vi "Monitor.vi"(8 "error in (no error)":errorcluster) -> ()   [LabVIEW 2015]
uses:
  <vilib>/Rock Robotics/Network Tables/NT Write Number.vi
  Utilities/MotorPositionGlobals.vi
  Utilities/GlobalVisionVars.vi
  MonitorGlobals.vi
  Utilities/ShiftGlobals.vi
  navx-mxp/labview/navX Library v2/navX Library v2.lvlib
panel:
  out "YRPHfH":T1
  out "Applied Throttle 2":dbl
  out "Applied Throttle":dbl
  out "Climber Current":dbl
  out "Climber Velocity":dbl
  out "Climber Position":dbl
  in  "Tab Control":enum32{"Position", "Vision Code", "Currents"}(tab)
  out "ArmMotor Encoder Position":dbl
  out "TensionerMotor Encoder Position":dbl
  out "WinchMotor Encoder Position":dbl
  out "WinchSetpoint":dbl
  out "TensionerSetpoint":dbl
  out "ArmSetpoint":dbl=195.0
  out "Manipulator Encoder":dbl
  out "Manipulator Setpoint":dbl
  out "Left Drive Encoder":dbl
  out "Right Drive Encoder":dbl
  out "Left Drive Velocity":dbl
  out "Right Drive Velocity":dbl
  out "Tensioner Limit Switch Pressed":bool
  out "Horizontal Gyro Angle":dbl
  out "LeftDriveError":dbl
  out "RightDriveError":dbl
  out "Heading vs Actual":dynamicdata(graph)
  out "TargetDistance":dbl
  out "Heading":dbl
  out "NumberOfParticles":i32
  out "OnTarget":bool
  out "Left1 Current":dbl
  out "Left2 Current":dbl
  out "Right1 Current":dbl
  out "Right2 Current":dbl
  out "Winch Current":dbl
  out "Arm Current":dbl
  out "Tensioner Current":dbl
  out "Manipulator Current":dbl
  out "all currents (A)":dbl[](array[numeric])
  out "Waveform Chart":dynamicdata(graph)
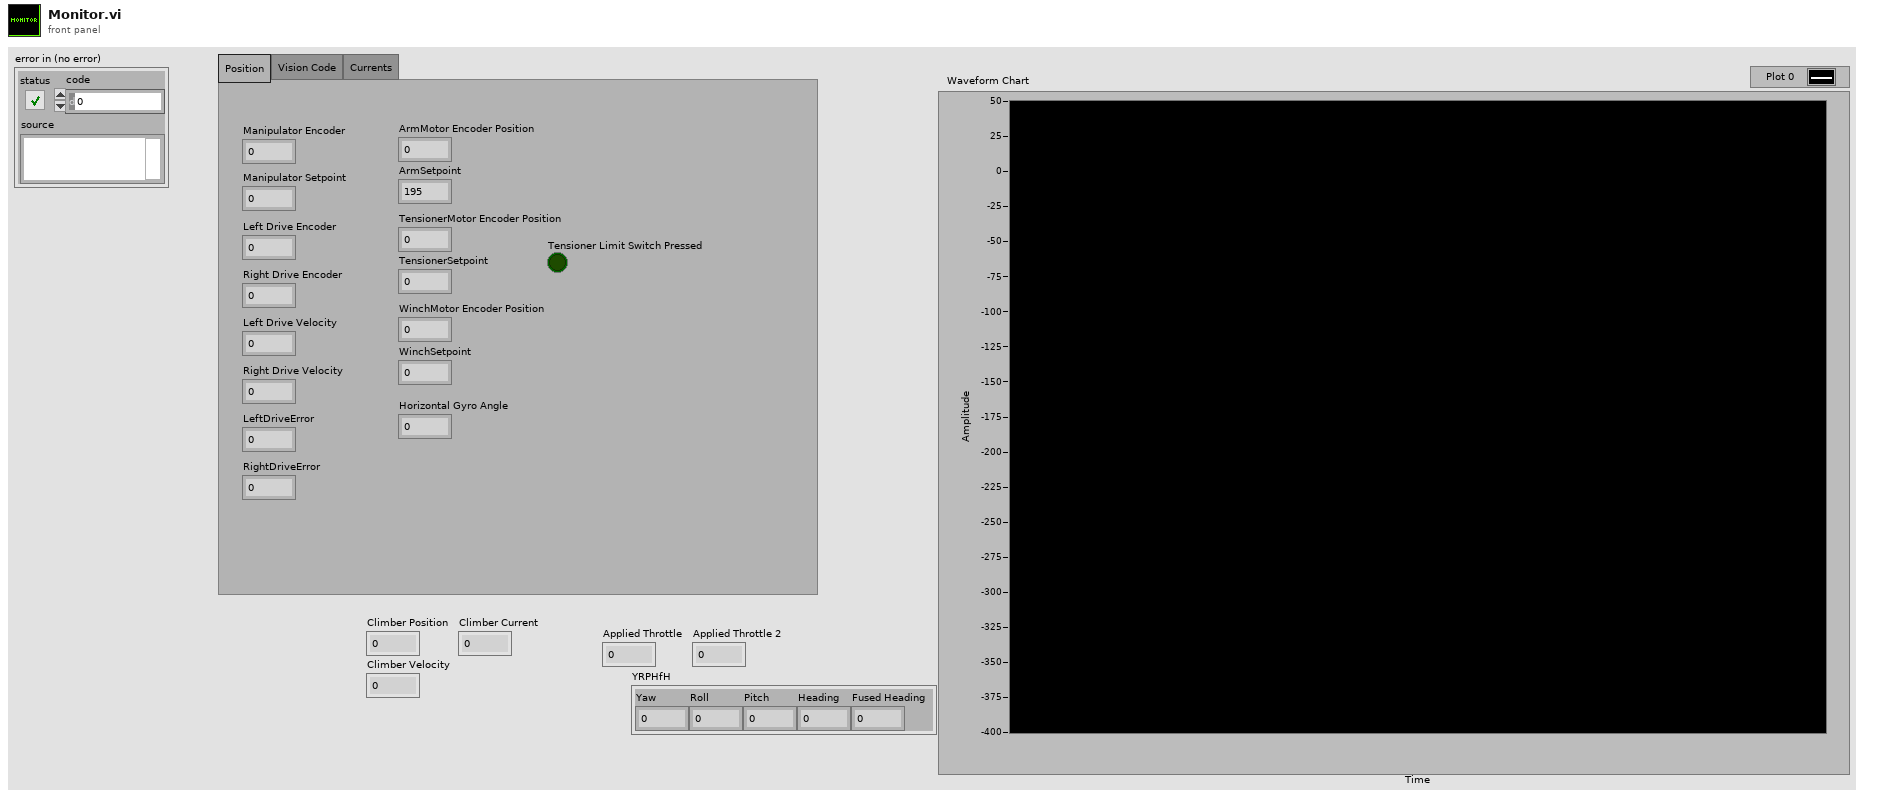
[diagram p1: front panel]
types:
  T1 = cluster{"Yaw":dbl, "Roll":dbl, "Pitch":dbl, "Heading":dbl, "Fused Heading":dbl}
  T2 = typedef "navX Library v2.lvlib/Z900_navX_DeviceTypeDef.ctl" = cluster{"Interface":cluster{"Protocol":T3, "Update Rate (4Hz-60Hz)":u8, "navX Open TypeDef":variant}, "Notify Packet":refnum<notifier>, "Loop VI Refnum":refnum<vi>, "Ready to Close Occurrence Refnum":refnum<k4>}
  T3 = typedef "navX Library v2.lvlib/Z900_navX_ProtocolTypeDef.ctl" = enum16{"SERIAL", "I2C", "SPI"}
  T4 = typedef "WPI_SwitchDevRef.ctl" = cluster{"DevStatus":errorcluster, "DIO Channel":T5, "CntIndex":T6, "Normally Closed":bool}
  T5 = typedef "FPGA_DIOChannel.ctl" = enum8{"DIO 0", "DIO 1", "DIO 2", "DIO 3", "DIO 4", "DIO 5", "DIO 6", "DIO 7", "DIO 8", "DIO 9", "DIO MXP 0", "DIO MXP 1", "DIO MXP 2", "DIO MXP 3", "DIO MXP 4", "DIO MXP 5", "DIO MXP 6", "DIO MXP 7", "DIO MXP 8", "DIO MXP 9", "DIO MXP 10", "DIO MXP 11", "DIO MXP 12", "DIO MXP 13", "DIO MXP 14", "DIO MXP 15", "Invalid"}
  T6 = typedef "FPGA_CounterCtrSystemIndex.ctl" = enum8{"Ctr 0", "Ctr 1", "Ctr 2", "Ctr 3", "Ctr 4", "Ctr 5", "Ctr 6", "Ctr 7", "Invalid"}
  T7 = typedef "WPI_MotorControlDeviceRef.ctl" = cluster{"DeviceStatus":errorcluster, "Type":T8, "PWM":cluster{"PWM Channel":T9, "DeadBand":T10}, "CAN":cluster{"Device Number":u8, "Control Mode":T11, "Semaphore":T12, "Max Vout":dbl, "TalonSRX Control Mode":T13}, "Invert":bool}
  T8 = typedef "WPI_MotorControlType.ctl" = enum16{"PWM", "CAN", "CANTalonSRX"}
  T9 = typedef "FPGA_DIOPWMChannel.ctl" = enum8{"PWM 0", "PWM 1", "PWM 2", "PWM 3", "PWM 4", "PWM 5", "PWM 6", "PWM 7", "PWM 8", "PWM 9", "PWM MXP 0", "PWM MXP 1", "PWM MXP 2", "PWM MXP 3", "PWM MXP 4", "PWM MXP 5", "PWM MXP 6", "PWM MXP 7", "PWM MXP 8", "PWM MXP 9", "Invalid"}
  T10 = typedef "WPI_PWMDeadband.ctl" = cluster{"Name":string, "maxPositivePwm":i32, "minPositivePwm":i32, "centerPwm":i32, "maxNegativePwm":i32, "minNegativePwm":i32, "angularRange":u16}
  T11 = typedef "WPI_CANJaguar_ControlMode.ctl" = enum8{"Percent VBus", "Current", "Speed", "Position", "Voltage"}
  T12 = typedef "Semaphore RefNum" = refnum<k1>
  T13 = typedef "WPI_CANTalonSRX_APIControlMode.ctl" = enum8{"Percent VBus", "Speed", "Position", "Slave", "Unchanged / Invalid", "Voltage Compensation", "Current", "Motion Profile"}
  T14 = typedef "WPI_GyroDevRef.ctl" = cluster{"DevStatus":errorcluster, "Analog Channel":T15, "Offset":dbl, "Gain (VoltsPerDegree/Second)":dbl, "Gyro Type":enum16{"Analog", "XRS450"}, "Handle":i32, "SPI Bus":T16, "Device Found":bool, "Sample Rate":dbl, "Calibrate On Open":bool}
  T15 = typedef "FPGA_AIChannel.ctl" = enum8{"AI 0", "AI 1", "AI 2", "AI 3", "AI MXP 0", "AI MXP 1", "AI MXP 2", "AI MXP 3", "Invalid"}
  T16 = typedef "spi_bus.ctl" = enum16{"SPI On-Board, CS0", "SPI On-Board, CS1", "SPI On-Board, CS2", "SPI On-Board, CS3", "SPI MXP", "Invalid"}
  T17 = typedef "WPI_CANTalonSRX_GlobalStatus.ctl" = cluster{"Applied Throttle":dbl, "Module Enabled":bool, "CAN Error":errorcluster, "Closed Loop Error":dbl, "Forward Limit Switch Closed":bool, "Reverse Limit Switch Closed":bool, "Sensor Position":dbl, "Sensor Velocity":dbl, "Current":dbl, "Sticky Fault - Over Temp":bool, "Sticky Fault - Under Voltage":bool, "Sticky Fault - Forward Limit":bool, "Sticky Fault - Reverse Limit":bool, "Sticky Fault - Forward Soft Limit":bool, "Sticky Fault - Reverse Soft Limit":bool, "Brake is Enabled":bool, "Encoder Position":dbl, "Encoder Velocity":dbl, "Encoder Index Count":dbl, "Encoder A Pin State":bool, "Encoder B Pin State":bool, "Encoder Index Pin State":bool, "Analog In":dbl, "Analog In Velocity":dbl, "Temperature (C)":dbl, "Battery Voltage":dbl, "Control 5 Is Supported":bool, "Current Profile Slot Select":dbl, "Pos Div 8":bool, "Vel Div 4":bool, "Pulse Width Position":i32, "Pulse Width Velocity":i32, "Pulse Width Rise To Rise (us)":i32, "Pulse Width Rise To Fall (us)":i32, "Mot Prof Active Is Under Run":bool, "Mot Prof Active Has Under Run":bool, "Mot Prof Active Is Last":bool, "Mot Prof Active Velocity Only":bool, "Mot Prof Active Is Valid":bool, "Mot Prof Buffer Is Full":bool, "Mot Prof Active Profile Slot Select":i32, "Mot Prof NextID":i32, "Mot Prof Count":i32, "Mot Prof Active Velocity":dbl, "Mot Prof Active Position":dbl, "Mot Prof Output Enable":i32}
  T18 = enum16{"open", "replace", "create", "open or create", "replace or create", "replace or create with confirmation"}
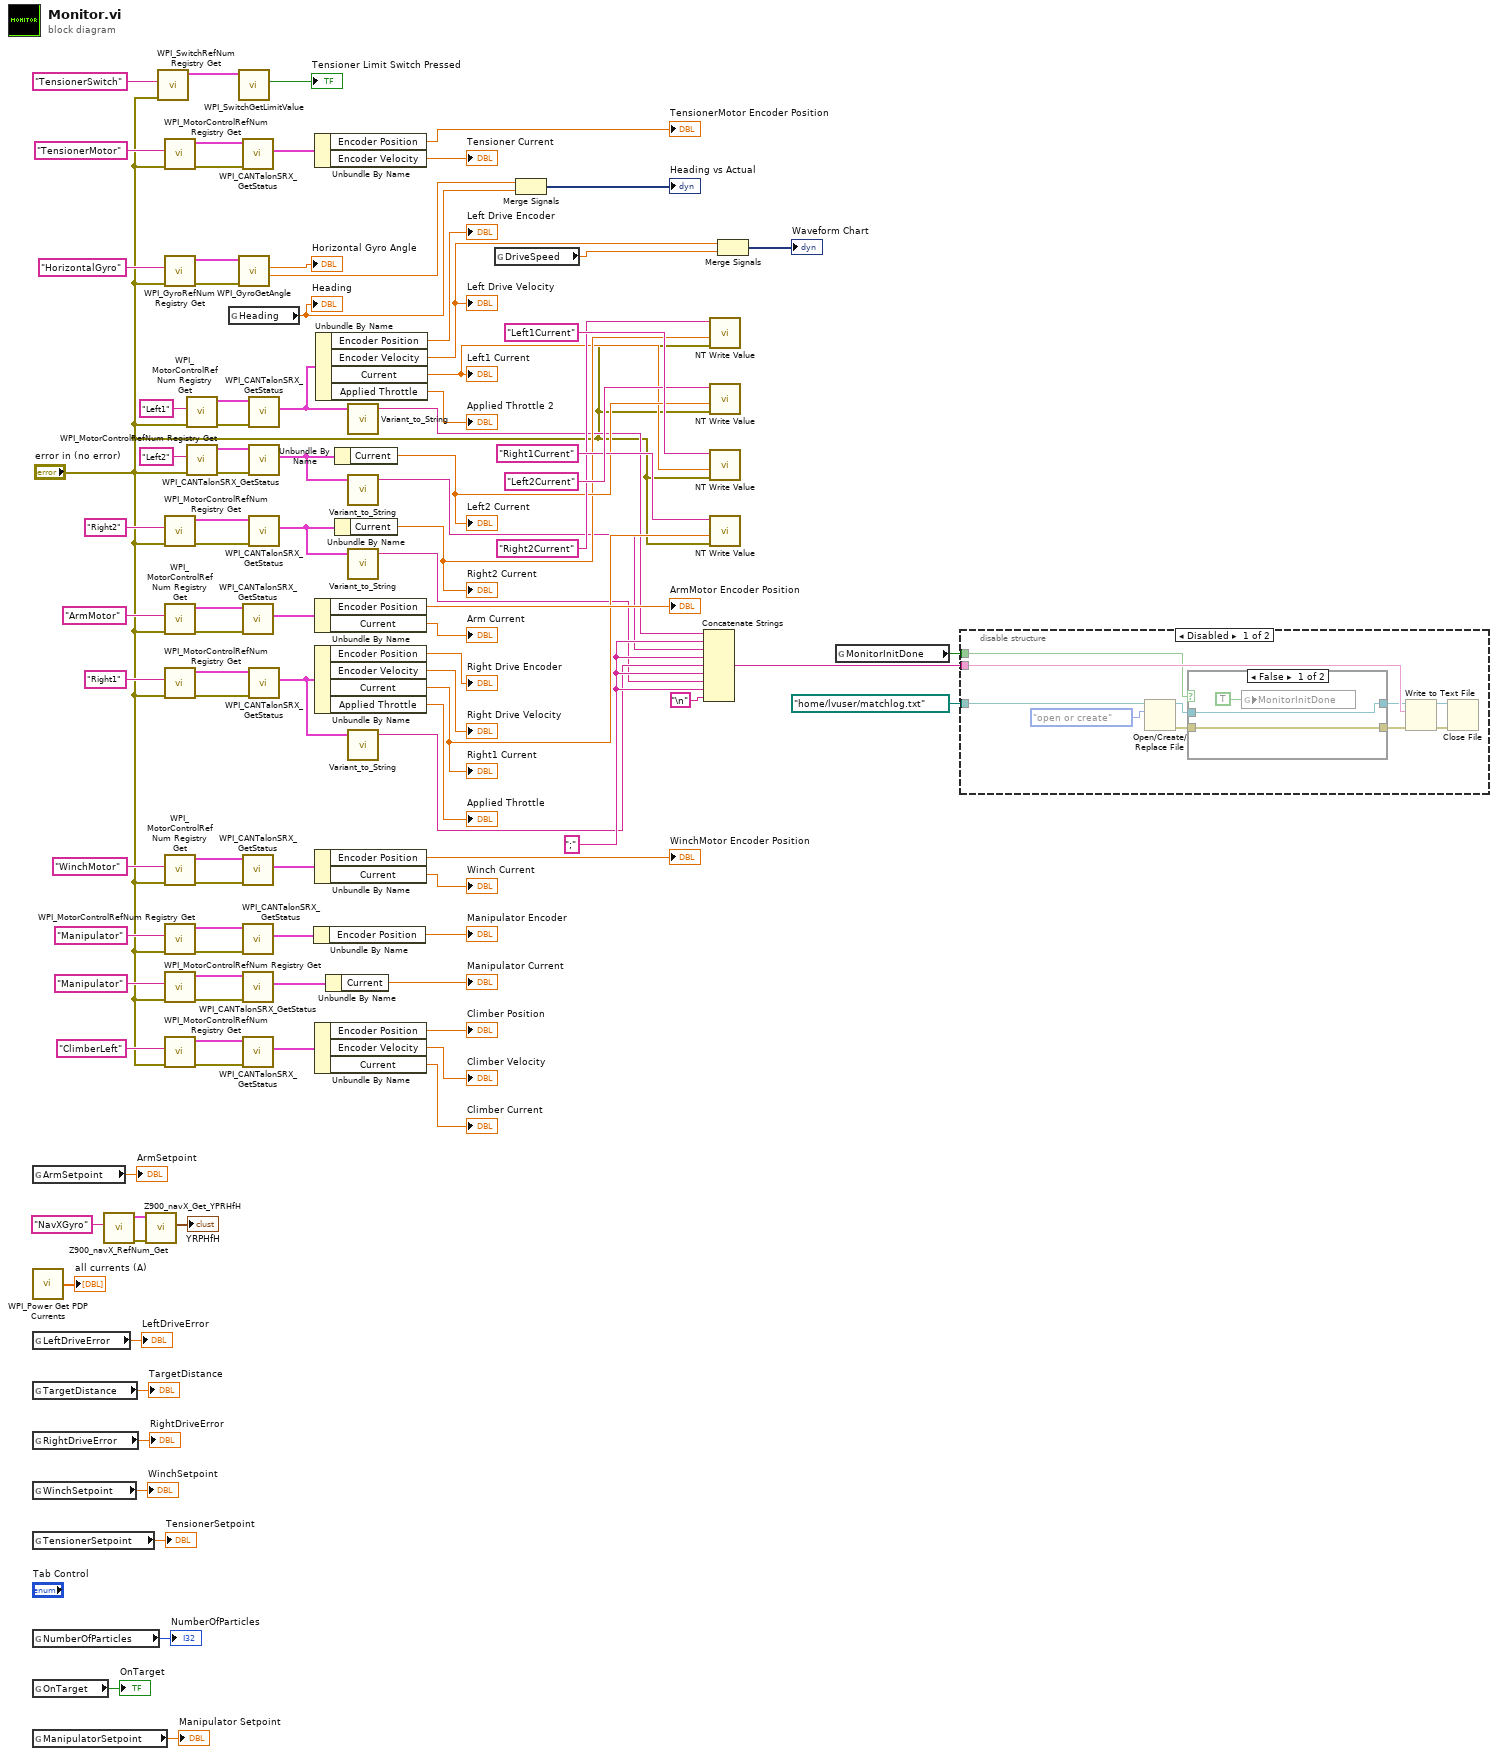
[diagram p0: block diagram]
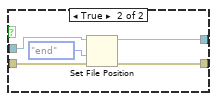
[diagram p2: hidden frame]
diagram:
  w27 = ";" ("string")
  n1 = global read "MotorPositionGlobals.vi" "ArmSetpoint"() -> (→"ArmSetpoint":dbl)
  n2 = call <vilib>:"WPI_Power Get PDP Currents.vi"() -> ("all currents (A)"=→"all currents (A)":dbl[])  [unwired: 13 in, 2 out]
  n3 = global read "MotorPositionGlobals.vi" "LeftDriveError"() -> (→"LeftDriveError":dbl)
  n4 = global read "GlobalVisionVars.vi" "TargetDistance"() -> (→"TargetDistance":dbl)
  n5 = global read "MotorPositionGlobals.vi" "RightDriveError"() -> (→"RightDriveError":dbl)
  n6 = global read "MotorPositionGlobals.vi" "WinchSetpoint"() -> (→"WinchSetpoint":dbl)
  n7 = global read "MotorPositionGlobals.vi" "TensionerSetpoint"() -> (→"TensionerSetpoint":dbl)
  n8 = global read "GlobalVisionVars.vi" "NumberOfParticles"() -> (→"NumberOfParticles":i32)
  n9 = global read "GlobalVisionVars.vi" "OnTarget"() -> (→"OnTarget":bool)
  n10 = global read "MotorPositionGlobals.vi" "ManipulatorSetpoint"() -> (→"Manipulator Setpoint":dbl)
  n11 = call "Z900_navX_RefNum_Get.vi"("refnum name"="NavXGyro") -> ("error out"=w3:errorcluster, "navX Device"=w4:T2)  [unwired: 9 in]
  n12 = call "Z900_navX_Get_YPRHfH.vi"("error in (no error)"=w3, "navX Device"=w4) -> ("YRPHfH"=→"YRPHfH":T1)  [unwired: 6 in, 3 out]
  n13 = call <vilib>:"WPI_SwitchRefNum Registry Get.vi"("error in (no error)"="error in (no error)", "refnum name"="TensionerSwitch") -> ("SwitchDevRef"=w86:T4)  [unwired: 8 in, 1 out]
  n14 = call <vilib>:"WPI_MotorControlRefNum Registry Get.vi"("error in (no error)"="error in (no error)", "refnum name"="TensionerMotor") -> ("error out"=w94:errorcluster, "MotorControlDevRef"=w93:T7)  [unwired: 8 in]
  n15 = call <vilib>:"WPI_GyroRefNum Registry Get.vi"("error in (no error)"="error in (no error)", "refnum name"="HorizontalGyro") -> ("error out"=w76:errorcluster, "GyroDevRef"=w77:T14)  [unwired: 8 in]
  n16 = call <vilib>:"WPI_MotorControlRefNum Registry Get.vi"("error in (no error)"="error in (no error)", "refnum name"="Right2") -> ("error out"=w59:errorcluster, "MotorControlDevRef"=w58:T7)  [unwired: 8 in]
  n17 = call <vilib>:"WPI_MotorControlRefNum Registry Get.vi"("error in (no error)"="error in (no error)", "refnum name"="ArmMotor") -> ("error out"=w98:errorcluster, "MotorControlDevRef"=w97:T7)  [unwired: 8 in]
  n18 = call <vilib>:"WPI_MotorControlRefNum Registry Get.vi"("error in (no error)"="error in (no error)", "refnum name"="Right1") -> ("error out"=w62:errorcluster, "MotorControlDevRef"=w63:T7)  [unwired: 8 in]
  n19 = call <vilib>:"WPI_MotorControlRefNum Registry Get.vi"("error in (no error)"="error in (no error)", "refnum name"="WinchMotor") -> ("error out"=w91:errorcluster, "MotorControlDevRef"=w90:T7)  [unwired: 8 in]
  n20 = call <vilib>:"WPI_MotorControlRefNum Registry Get.vi"("error in (no error)"="error in (no error)", "refnum name"="Manipulator") -> ("error out"=w70:errorcluster, "MotorControlDevRef"=w69:T7)  [unwired: 8 in]
  n21 = call <vilib>:"WPI_MotorControlRefNum Registry Get.vi"("error in (no error)"="error in (no error)", "refnum name"="Manipulator") -> ("error out"=w52:errorcluster, "MotorControlDevRef"=w53:T7)  [unwired: 8 in]
  n22 = call <vilib>:"WPI_MotorControlRefNum Registry Get.vi"("error in (no error)"="error in (no error)", "refnum name"="ClimberLeft") -> ("error out"=w15:errorcluster, "MotorControlDevRef"=w14:T7)  [unwired: 8 in]
  n23 = call <vilib>:"WPI_MotorControlRefNum Registry Get.vi"("error in (no error)"="error in (no error)", "refnum name"="Left1") -> ("error out"=w82:errorcluster, "MotorControlDevRef"=w81:T7)  [unwired: 8 in]
  n24 = call <vilib>:"WPI_MotorControlRefNum Registry Get.vi"("error in (no error)"="error in (no error)", "refnum name"="Left2") -> ("error out"=w65:errorcluster, "MotorControlDevRef"=w64:T7)  [unwired: 8 in]
  n25 = global read "GlobalVisionVars.vi" "Heading"() -> (w34:dbl)
  "Heading" <- w34
  n26 = call <vilib>:"WPI_SwitchGetLimitValue.vi"("SwitchDevRef"=w86) -> ("Switch Pressed"=→"Tensioner Limit Switch Pressed":bool)  [unwired: 8 in, 2 out]
  n27 = call <vilib>:"WPI_GyroGetAngle.vi"("error in"=w76, "GyroDevRef"=w77) -> ("Angular Rate"=w36:dbl, "Angle"=→"Horizontal Gyro Angle":dbl)  [unwired: 5 in, 3 out]
  n28 = call <vilib>:"WPI_CANTalonSRX_GetStatus.vi"("error in (no error)"=w94, "CAN Talon SRX Ref"=w93) -> ("Talon SRX Status"=w95:T17)  [unwired: 7 in, 2 out]
  n29 = call <vilib>:"WPI_CANTalonSRX_GetStatus.vi"("error in (no error)"=w98, "CAN Talon SRX Ref"=w97) -> ("Talon SRX Status"=w96:T17)  [unwired: 7 in, 2 out]
  n30 = call <vilib>:"WPI_CANTalonSRX_GetStatus.vi"("error in (no error)"=w91, "CAN Talon SRX Ref"=w90) -> ("Talon SRX Status"=w92:T17)  [unwired: 7 in, 2 out]
  n31 = call <vilib>:"WPI_CANTalonSRX_GetStatus.vi"("error in (no error)"=w70, "CAN Talon SRX Ref"=w69) -> ("Talon SRX Status"=w68:T17)  [unwired: 7 in, 2 out]
  n32 = call <vilib>:"WPI_CANTalonSRX_GetStatus.vi"("error in (no error)"=w52, "CAN Talon SRX Ref"=w53) -> ("Talon SRX Status"=w51:T17)  [unwired: 7 in, 2 out]
  n33 = call <vilib>:"WPI_CANTalonSRX_GetStatus.vi"("error in (no error)"=w15, "CAN Talon SRX Ref"=w14) -> ("Talon SRX Status"=w12:T17)  [unwired: 7 in, 2 out]
  n34 = call <vilib>:"WPI_CANTalonSRX_GetStatus.vi"("error in (no error)"=w82, "CAN Talon SRX Ref"=w81) -> ("Talon SRX Status"=w25:T17)  [unwired: 7 in, 2 out]
  n35 = call <vilib>:"WPI_CANTalonSRX_GetStatus.vi"("error in (no error)"=w65, "CAN Talon SRX Ref"=w64) -> ("Talon SRX Status"=w30:T17)  [unwired: 7 in, 2 out]
  n36 = call <vilib>:"WPI_CANTalonSRX_GetStatus.vi"("error in (no error)"=w59, "CAN Talon SRX Ref"=w58) -> ("Talon SRX Status"=w28:T17)  [unwired: 7 in, 2 out]
  n37 = call <vilib>:"WPI_CANTalonSRX_GetStatus.vi"("error in (no error)"=w62, "CAN Talon SRX Ref"=w63) -> ("Talon SRX Status"=w29:T17)  [unwired: 7 in, 2 out]
  n38 = Unbundle By Name(w68) -> ("Encoder Position"=→"Manipulator Encoder":dbl)
  n39 = Unbundle By Name(w95) -> ("Encoder Position"=→"TensionerMotor Encoder Position":dbl, "Encoder Velocity"=→"Tensioner Current":dbl)
  n40 = Unbundle By Name(w96) -> ("Encoder Position"=→"ArmMotor Encoder Position":dbl, "Current"=→"Arm Current":dbl)
  n41 = Unbundle By Name(w29) -> ("Encoder Position"=→"Right Drive Encoder":dbl, "Encoder Velocity"=→"Right Drive Velocity":dbl, "Current"=w31:dbl, "Applied Throttle"=→"Applied Throttle":dbl)
  "Right1 Current" <- w31
  n42 = Unbundle By Name(w92) -> ("Encoder Position"=→"WinchMotor Encoder Position":dbl, "Current"=→"Winch Current":dbl)
  n43 = Unbundle By Name(w12) -> ("Encoder Position"=→"Climber Position":dbl, "Encoder Velocity"=→"Climber Velocity":dbl, "Current"=→"Climber Current":dbl)
  n44 = Unbundle By Name(w25) -> ("Encoder Position"=→"Left Drive Encoder":dbl, "Encoder Velocity"=w8:dbl, "Current"=w26:dbl, "Applied Throttle"=→"Applied Throttle 2":dbl)
  "Left Drive Velocity" <- w8
  "Left1 Current" <- w26
  n45 = Unbundle By Name(w51) -> ("Current"=→"Manipulator Current":dbl)
  n46 = Unbundle By Name(w30) -> ("Current"=w44:dbl)
  "Left2 Current" <- w44
  n47 = Unbundle By Name(w28) -> ("Current"=w43:dbl)
  "Right2 Current" <- w43
  n48 = call "Variant_to_String.vi"("Variant"=w25) -> ("String"=w24:string)  [unwired: 3 in, 1 out]
  n49 = call "Variant_to_String.vi"("Variant"=w30) -> ("String"=w23:string)  [unwired: 3 in, 1 out]
  n50 = call "Variant_to_String.vi"("Variant"=w28) -> ("String"=w21:string)  [unwired: 3 in, 1 out]
  n51 = call "Variant_to_String.vi"("Variant"=w29) -> ("String"=w22:string)  [unwired: 3 in, 1 out]
  n52 = global read "ShiftGlobals.vi" "DriveSpeed"() -> (w7:dbl)
  n53 = Merge Signals(w36, w34) -> (→"Heading vs Actual":dynamicdata)
  n54 = Concatenate Strings(w24, w27, w23, w27, w22, w27, w21, w27, "\n") -> (w19:string)
  n55 = call-poly <vilib>:"NT Write Value.vi"("error in"="error in (no error)", "Numeric"=w43, "Name"="Right2Current") -> ()  [unwired: 8 in, 1 out]
  n56 = call-poly <vilib>:"NT Write Value.vi"("error in"="error in (no error)", "Numeric"=w44, "Name"="Left2Current") -> ()  [unwired: 8 in, 1 out]
  n57 = call-poly <vilib>:"NT Write Value.vi"("error in"="error in (no error)", "Numeric"=w26, "Name"="Left1Current") -> ()  [unwired: 8 in, 1 out]
  n58 = call-poly <vilib>:"NT Write Value.vi"("error in"="error in (no error)", "Numeric"=w31, "Name"="Right1Current") -> ()  [unwired: 8 in, 1 out]
  n59 = Merge Signals(w8, w7) -> (→"Waveform Chart":dynamicdata)
  n60 = global read "MonitorGlobals.vi" "MonitorInitDone"() -> (w17:bool)
  n61 = disable-structure shown="Disabled" {
    disable-tunnel: path "/home/lvuser/matchlog.txt" ("file path (use dialog)") -> [w111 _]
    disable-tunnel: w19 -> [w110 _]
    disable-tunnel: w17 -> [w109 _]
    frame Disabled {
      n62 = Open/Create/Replace File(file path (use dialog)=w111, operation (0:open)=T18."open or create") -> (refnum out=w108:refnum<file>, error out=w107:errorcluster)  [unwired: 4 in, 1 out]
      n63 = case shown="False" w109 {
        tunnel: w108 -> [w114 w119]
        tunnel: w107 -> [w113 w117]
        tunnel: [w113 w116] -> w106
        tunnel: [w114 w115] -> w105
        frame False {
          n64 = global write "MonitorGlobals.vi" "MonitorInitDone"(TRUE ("InitDone")) -> ()
        }
        frame True {
          n65 = Set File Position(refnum=w119, from (0:start)=enum16{"start", "end", "current"}."end", error in=w117) -> (refnum out=w115:refnum<file>, error out=w116:errorcluster)  [unwired: 1 in]
        }
      }
      n66 = Write to Text File(file (use dialog)=w105, text=w110, error in=w106) -> (refnum out=w104:refnum<file>, error out=w103:errorcluster)  [unwired: 1 in, 1 out]
      n67 = Close File(refnum=w104, error in=w103) -> ()  [unwired: 2 out]
    }
    frame Enabled {
    }
  }
